vi "ProfilerTest.vi"() -> ()   [LabVIEW 2014] (continued)
    n15 = Index Array(array=w77, index #1=w67, index #2=w82) -> (element #1=w65:T8, element #2=w81:T8)
    n16 = Unbundle By Name(w58) -> ("Velocity"=w72:dbl)
    n17 = Unbundle By Name(w65) -> ("Velocity"=w79:dbl)
    n18 = Unbundle By Name(w70) -> ("Time"=w73:dbl)
    n19 = Unbundle By Name(w81) -> ("Time"=w78:dbl)
    n20 = Unbundle(w65) -> ("Time"=w64:dbl, "Velocity"=w63:dbl)  [unwired: 2 out]
    n21 = Bundle("Time"=w64, "Velocity"=w63) -> (w62:cluster{"Time":dbl, "Velocity":dbl})  [unwired: 1 in]
    n22 = Unbundle(w58) -> ("Time"=w60:dbl, "Velocity"=w61:dbl)  [unwired: 2 out]
    n23 = Bundle By Name(cluster=w80, "delVelocity"=w79, "Time"=w78) -> (w76:cluster{"Time":dbl, "delVelocity":dbl})
    n24 = Bundle By Name(cluster=w71, "Velocity"=w72, "Time"=w73) -> (w74:cluster{"Time":dbl, "Velocity":dbl})
    n25 = Bundle("Time"=w60, "Velocity"=w61) -> (w59:cluster{"Time":dbl, "Velocity":dbl})  [unwired: 1 in]
    n26 = Build Array(w59, w74) -> (w66:cluster{"Time":dbl, "Velocity":dbl}[])
    n27 = Build Array(w62, w76) -> (w75:cluster{"Time":dbl, "delVelocity":dbl}[])
  }
  n28 = call "Vel2Accel.vi"("MaxJerk"="MaxJerk", "Acceleration Max"="Acceleration Max", "Velocities"=w15) -> ("AccelParams"=w12:T4)  [unwired: 8 in]
  "xAccel" <- w12
  n29 = call "Vel2Accel.vi"("MaxJerk"="MaxJerk", "Acceleration Max"="Acceleration Max", "Velocities"=w14) -> ("AccelParams"=w10:T4)  [unwired: 8 in]
  "yAccel" <- w10
  n30 = for {
    tunnel: w12 -> [w84] mode=indexing
    tunnel: [w84] -> w11 mode=indexing if=w83
    n31 = Unbundle By Name(w84) -> ("A"=w85:dbl)
    n32 = Not Equal To 0?(x=w85) -> (x != 0?=w83:bool)
  }
  n33 = for {
    tunnel: w10 -> [w87] mode=indexing
    tunnel: [w87] -> w9 mode=indexing if=w86
    n34 = Unbundle By Name(w87) -> ("A"=w88:dbl)
    n35 = Not Equal To 0?(x=w88) -> (x != 0?=w86:bool)
  }
  n36 = Bundle(w46) -> (w38:T9)  [unwired: 1 in]
  n37 = Bundle(w45) -> (w37:cluster{cluster{"Time":dbl, "Velocity":dbl}[]})  [unwired: 1 in]
  n38 = call "Accel2Pos_RatePoints.vi"("Points"="Points", "Rate (hz)"="Rate (hz)", "Start (s)"="Start (s)", "Accel"=w9) -> ("Times"=w19:dbl[], "Velocities"=w28:dbl[], "Positions"=w2:dbl[])  [unwired: 5 in]
  n39 = call "Accel2Pos_RatePoints.vi"("Points"="Points", "Rate (hz)"="Rate (hz)", "Start (s)"="Start (s)", "Accel"=w11) -> ("Times"=w20:dbl[], "Velocities"=w29:dbl[], "Positions"=w16:dbl[])  [unwired: 5 in]
  n40 = Array Size(array=w2) -> (size(s)=→"SizeOut":i32)
  n41 = Build Cluster Array(w16, w2) -> (w18:cluster{dbl, dbl}[])
  n42 = Bundle(w18) -> (w17:cluster{cluster{dbl, dbl}[]})  [unwired: 1 in]
  n43 = Build Array(w22, w17) -> (→"XY Graph":T5)
  n44 = for {
    tunnel: w12 -> [w132] mode=indexing
    tunnel: [w111] -> w43 mode=concatenating
    tunnel: w10 -> [w90] mode=indexing
    tunnel: [w89] -> w41 mode=concatenating
    n45 = Unbundle By Name(w90) -> ("End"=w107:dbl, "Start"=w106:dbl, "A"=w92:dbl, "B"=w93:dbl, "Center"=w94:dbl)
    n46 = Unbundle By Name(w132) -> ("End"=w115:dbl, "Start"=w116:dbl, "A"=w130:dbl, "B"=w129:dbl, "Center"=w128:dbl)
    n47 = Number To Fractional String(number=w92) -> (F-format string=w95:string)  [unwired: 3 in]
    n48 = Number To Fractional String(number=w93) -> (F-format string=w97:string)  [unwired: 3 in]
    n49 = Number To Fractional String(number=w94) -> (F-format string=w100:string)  [unwired: 3 in]
    n50 = Number To Fractional String(number=w130) -> (F-format string=w127:string)  [unwired: 3 in]
    n51 = Number To Fractional String(number=w129) -> (F-format string=w125:string)  [unwired: 3 in]
    n52 = Number To Fractional String(number=w128) -> (F-format string=w122:string)  [unwired: 3 in]
    n53 = Bundle("C", w100) -> (w103:cluster{string, string})  [unwired: 1 in]
    n54 = Bundle("C", w122) -> (w119:cluster{string, string})  [unwired: 1 in]
    n55 = Bundle("A", w95) -> (w101:cluster{string, string})  [unwired: 1 in]
    n56 = Bundle("B", w97) -> (w102:cluster{string, string})  [unwired: 1 in]
    n57 = Bundle("A", w127) -> (w121:cluster{string, string})  [unwired: 1 in]
    n58 = Bundle("B", w125) -> (w120:cluster{string, string})  [unwired: 1 in]
    n59 = Build Array(w101, w102, w103) -> (w104:cluster{string, string}[])
    n60 = call <vilib>:"Substitute Variables.vi"("Substitution Rules"=w104, "original formula"="A*cos(B*(x-C))^2") -> ("formula after substitution"=w105:string)  [unwired: 1 in, 1 out]
    n61 = Build Array(w121, w120, w119) -> (w118:cluster{string, string}[])
    n62 = call <vilib>:"Substitute Variables.vi"("Substitution Rules"=w118, "original formula"="A*cos(B*(x-C))^2") -> ("formula after substitution"=w117:string)  [unwired: 1 in, 1 out]
    n63 = call <vilib>:"Eval y=f(x) Optimal Step.vi"("number of points"=u32 100, "formula"=w105, "end"=w107, "start"=w106) -> ("Y Values"=w110:dbl[], "X Values"=w109:dbl[])  [unwired: 1 in, 2 out]
    n64 = call <vilib>:"Eval y=f(x) Optimal Step.vi"("number of points"=u32 100, "formula"=w117, "end"=w115, "start"=w116) -> ("Y Values"=w112:dbl[], "X Values"=w113:dbl[])  [unwired: 1 in, 2 out]
    n65 = Build Cluster Array(w109, w110) -> (w89:cluster{dbl, dbl}[])
    n66 = Build Cluster Array(w113, w112) -> (w111:cluster{dbl, dbl}[])
  }
  n67 = Bundle(w43) -> (w42:cluster{cluster{dbl, dbl}[]})  [unwired: 1 in]
  n68 = Bundle(w41) -> (w40:cluster{cluster{dbl, dbl}[]})  [unwired: 1 in]
  n69 = Build Cluster Array(w20, w29) -> (w27:cluster{dbl, dbl}[])
  n70 = Build Cluster Array(w19, w28) -> (w26:cluster{dbl, dbl}[])
  n71 = Build Array(w42, w40) -> (→"Accel":cluster{cluster{dbl, dbl}[]}[])
  n72 = Build Cluster Array(w20, w16) -> (w33:cluster{dbl, dbl}[])
  n73 = Build Cluster Array(w19, w2) -> (w31:cluster{dbl, dbl}[])
  n74 = Bundle(w27) -> (w25:cluster{cluster{dbl, dbl}[]})  [unwired: 1 in]
  n75 = Bundle(w26) -> (w24:cluster{cluster{dbl, dbl}[]})  [unwired: 1 in]
  n76 = Bundle(w33) -> (w32:cluster{cluster{dbl, dbl}[]})  [unwired: 1 in]
  n77 = Bundle(w31) -> (w30:cluster{cluster{dbl, dbl}[]})  [unwired: 1 in]
  n78 = Build Array(w38, w37, w25, w24) -> (→"VelocityProfile":cluster{cluster{"Time":dbl, "Velocity":dbl}[]}[])
  n79 = Build Array(w32, w30) -> (→"PositionProfile":cluster{cluster{dbl, dbl}[]}[])
